vi "Translator.vi"(0 "Input":variant, 11 "error in (no error)":errorcluster) -> (4 "Output":variant, 15 "error out":errorcluster)   [LabVIEW 2014, in "Complex Numbers.lvlib"]
doc: "An example of how to create the Translator to convert the LabVIEW VIs to Arduino C code."
uses:
  <vilib>/Aledyne-TSXperts/Arduino Compatible Compiler for LabVIEW/addons/Complex Numbers/Complex Numbers.lvlib
panel:
  out "Outputs":string[](array[string])
  out "Inputs":string[](array[string])
  out "Output Datatypes":string[](array[string])
  out "Input Datatypes":string[](array[string])
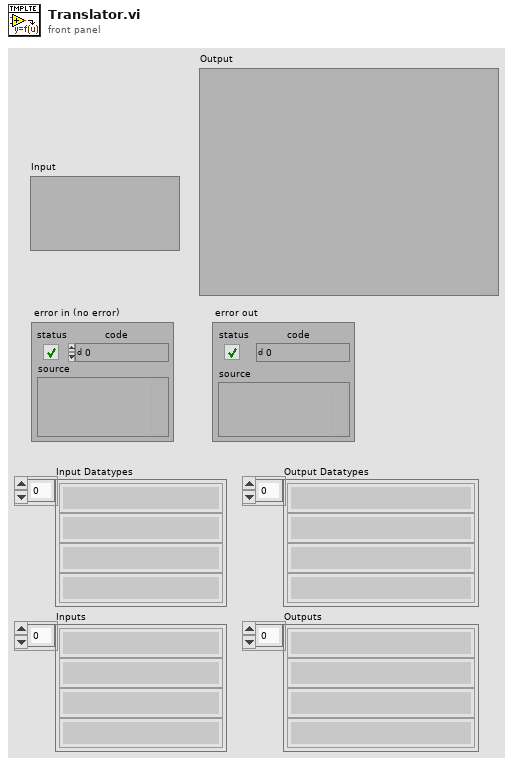
[diagram p1: front panel]
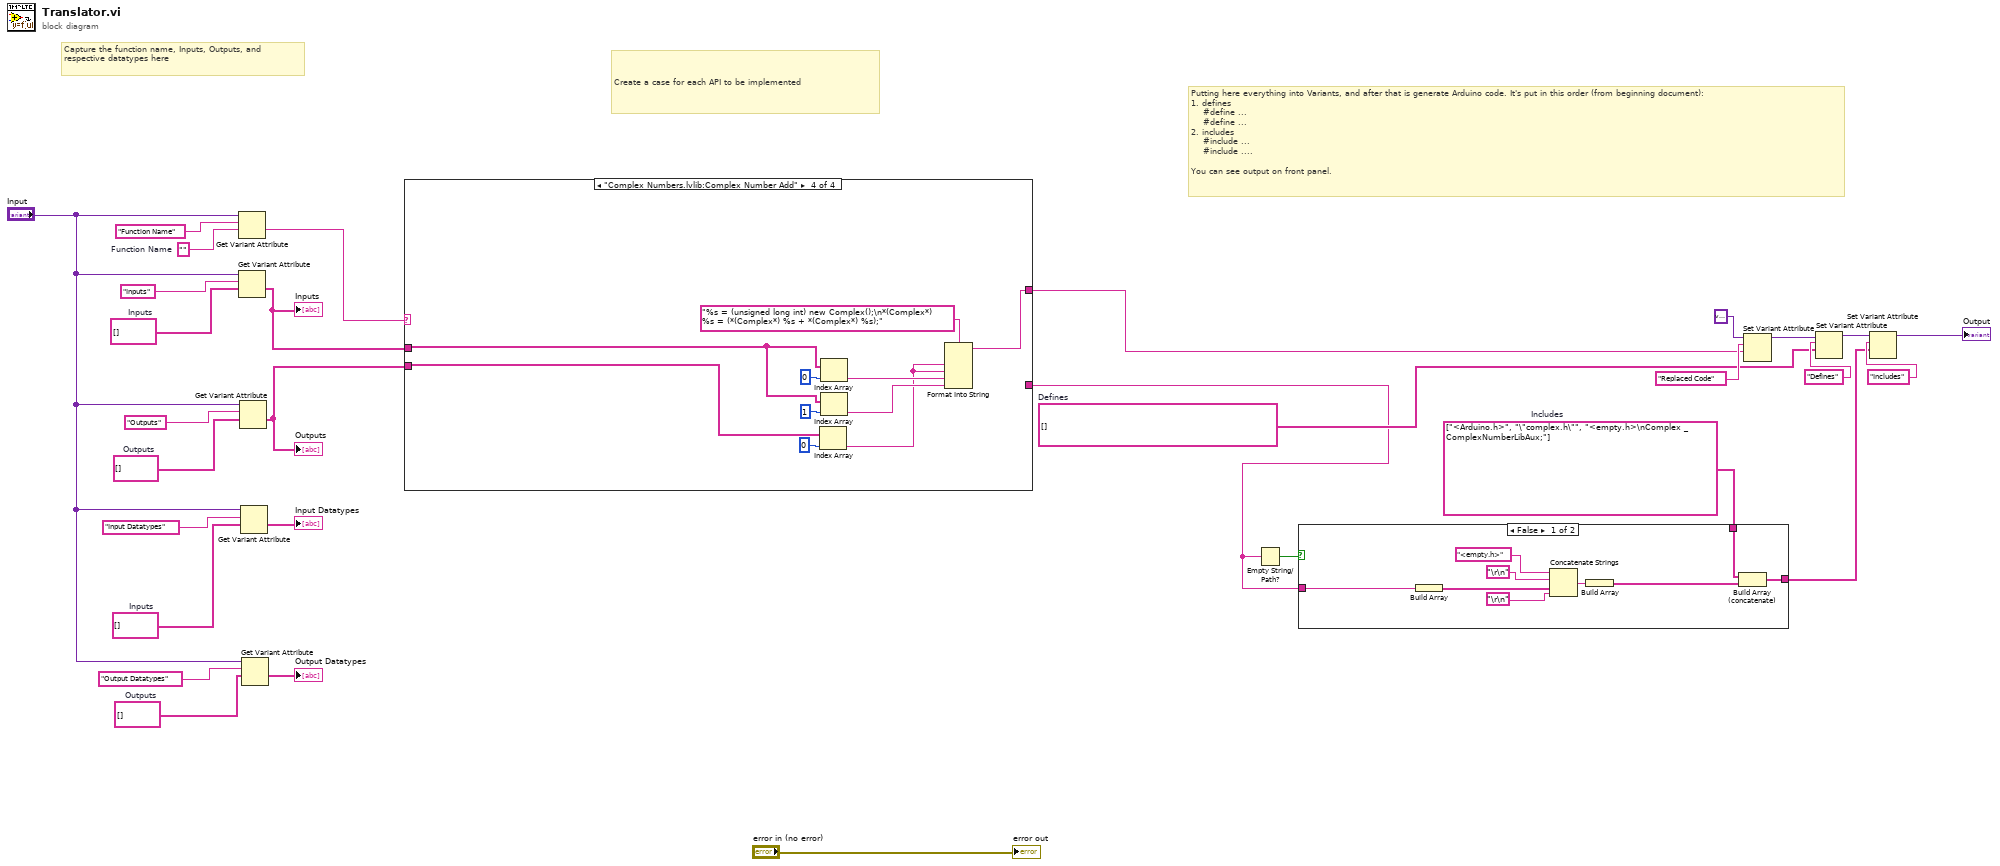
[diagram p0: block diagram]
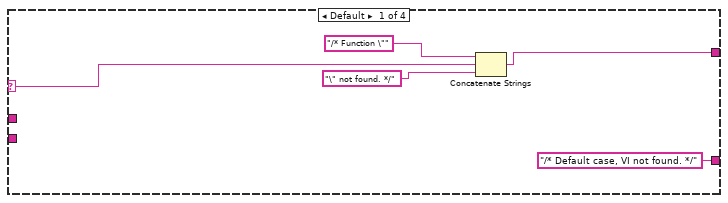
[diagram p3: hidden frame]
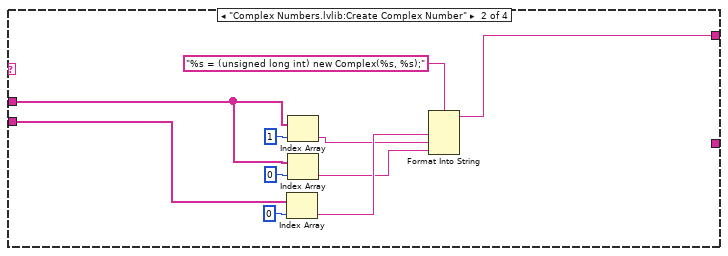
[diagram p4: hidden frame]
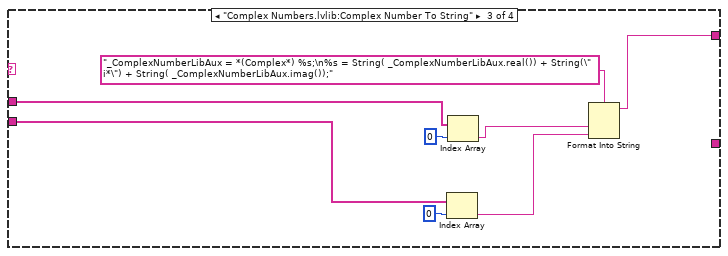
[diagram p5: hidden frame]
diagram:
  w4 = string[] []  # Defines
  w19 = string[] []  # Outputs
  w20 = string[] []  # Inputs
  w1 = string[] ["<Arduino.h>", "\"complex.h\"", "<empty.h>\nComplex _ComplexNumberLibAux;"]  # Includes
  w26 = string[] []  # Outputs
  w27 = string[] []  # Inputs
  w28 = ""  # Function Name
  # "Capture the function name, Inputs, Outputs, and respective datatypes here"
  # "Putting here everything into Variants, and after that is generate Arduino code. It's put in this order (from beginning document):\n1. defines\n    #define ...\n    #define ...\n2. includes\n    #include ...\n    #include ....\n\nYou can see output on front panel."
  # "Create a case for each API to be implemented"
  n1 = Get Variant Attribute(Variant="Input", name="Function Name", default value (empty Variant)=w28) -> (value=w10:string)  [unwired: 1 in, 3 out]
  n2 = Get Variant Attribute(Variant="Input", name="Inputs", default value (empty Variant)=w27) -> (value=w9:string[])  [unwired: 1 in, 3 out]
  "Inputs" <- w9
  n3 = Get Variant Attribute(Variant="Input", name="Outputs", default value (empty Variant)=w26) -> (value=w8:string[])  [unwired: 1 in, 3 out]
  "Outputs" <- w8
  n4 = Get Variant Attribute(Variant="Input", name="Input Datatypes", default value (empty Variant)=w20) -> (value=→"Input Datatypes":string[])  [unwired: 1 in, 3 out]
  n5 = Get Variant Attribute(Variant="Input", name="Output Datatypes", default value (empty Variant)=w19) -> (value=→"Output Datatypes":string[])  [unwired: 1 in, 3 out]
  n6 = case shown="\"Complex Numbers.lvlib:Complex Number Add\"" w10 {
    selector: w10 -> [w33 _ _ _]
    tunnel: w9 -> [_ w38 w47 w57]
    tunnel: w8 -> [_ w42 w50 w59]
    tunnel: [w31 w41 w49 w55] -> w7
    tunnel: ["/* Default case, VI not found. */" ("name") _ _ _] -> w3
    frame Default {
      n7 = Concatenate Strings("/* Function \"" ("string"), w33, "\" not found. */" ("string")) -> (w31:string)
    }
    frame "Complex Numbers.lvlib:Create Complex Number" {
      n8 = Index Array(array=w42, index=0) -> (element=w44:string)
      n9 = Index Array(array=w38, index=1) -> (element=w37:string)
      n10 = Index Array(array=w38, index=0) -> (element=w36:string)
      n11 = Format Into String(format string="%s = (unsigned long int) new Complex(%s, %s);", w44, w37, w36) -> (resulting string=w41:string)  [unwired: 2 in, 1 out]
    }
    frame "Complex Numbers.lvlib:Complex Number To String" {
      n12 = Index Array(array=w50, index=0) -> (element=w52:string)
      n13 = Index Array(array=w47, index=0) -> (element=w46:string)
      n14 = Format Into String(format string="_ComplexNumberLibAux = *(Complex*) %s;\n%s = String( _ComplexNumberLibAux.real()) + String(\" i*\") + String( _ComplexNumberLibAux.imag());", w46, w52) -> (resulting string=w49:string)  [unwired: 2 in, 1 out]
    }
    frame "Complex Numbers.lvlib:Complex Number Add" {
      n15 = Index Array(array=w59, index=0) -> (element=w54:string)
      n16 = Index Array(array=w57, index=0) -> (element=w63:string)
      n17 = Index Array(array=w57, index=1) -> (element=w56:string)
      n18 = Format Into String(format string="%s = (unsigned long int) new Complex();\n*(Complex*) %s = (*(Complex*) %s + *(Complex*) %s);", w54, w54, w63, w56) -> (resulting string=w55:string)  [unwired: 2 in, 1 out]
    }
  }
  n19 = Empty String/Path?(string/path=w3) -> (empty?=w5:bool)
  n20 = case shown="False" w5 {
    tunnel: w3 -> [w72 _]
    tunnel: [w65 w73] -> w2
    tunnel: w1 -> [w64 w73]
    frame False {
      n21 = Build Array(w72) -> (w66:string[])
      n22 = Concatenate Strings("<empty.h>" ("string"), "\r\n", w66, "\r\n") -> (w67:string)
      n23 = Build Array(w67) -> (w71:string[])
      n24 = Build Array (concatenate)(w64, w71) -> (w65:string[])
    }
    frame True {
    }
  }
  n25 = Set Variant Attribute(Variant=variant ("variant"), name="Replaced Code", value=w7) -> (Variant out=w13:variant)  [unwired: 1 in, 2 out]
  n26 = Set Variant Attribute(Variant=w13, name="Defines", value=w4) -> (Variant out=w12:variant)  [unwired: 1 in, 2 out]
  n27 = Set Variant Attribute(Variant=w12, name="Includes", value=w2) -> (Variant out=→"Output":variant)  [unwired: 1 in, 2 out]
  "error out" <- "error in (no error)"
